vi "SET_SHOOTER_ANGLE.vi"(10 "argv":string[](array[string]), 11 "args":u8) -> ()   [LabVIEW 2015]
uses:
  Team Code/Robot Global Data.vi
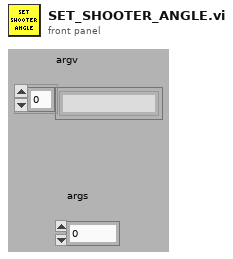
[diagram p1: front panel]
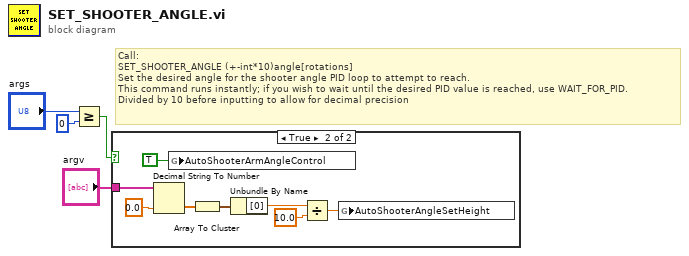
[diagram p0: block diagram]
diagram:
  # "Call:\nSET_SHOOTER_ANGLE (+-int*10)angle[rotations]\nSet the desired angle for the shooter angle PID loop to attempt to reach.\nThis command runs instantly; if you wish to wait until the desired PID value is reached, use WAIT_FOR_PID.\nDivided by 10 before inputting to allow for decimal precision"
  n1 = Greater Or Equal?(x="args", y=u8 0) -> (x >= y?=w4:bool)
  n2 = case shown="True" w4 {
    tunnel: "argv" -> [_ w12]
    frame False {
    }
    frame True {
      n3 = Decimal String To Number(string=w12, default (0L)=0.0 ("default (0 I32)")) -> (number=w10:dbl[])  [unwired: 2 out]
      n4 = global write "Robot Global Data.vi" "AutoShooterArmAngleControl"(TRUE ("AutoArmControl")) -> ()
      n5 = Array To Cluster(array=w10) -> (cluster=w9:cluster{"[0]":dbl, "[1]":dbl})
      n6 = Unbundle By Name(w9) -> ("[0]"=w7:dbl)
      n7 = Divide(x=w7, y=10.0) -> (x/y=w6:dbl)
      n8 = global write "Robot Global Data.vi" "AutoShooterAngleSetHeight"(w6) -> ()
    }
  }
